vi "GetModuleReport (SubVI).vi"(8 "error in (no error)":errorcluster, 9 "Calibrated positions of fiducials [mm]":dbl[][](array[numeric]), 10 "ith Module":i32, 11 "Module Progress Report in":T1(array[cluster])) -> (0 "error out":errorcluster, 1 "MyCorners":dbl[][](array[numeric]), 2 "Array of ith module cluster fiducial mark positions":cluster{"X":dbl, "Y":dbl, "Z":dbl}[](array[cluster]), 3 "Module Progress Report out":T1(array[cluster]))   [LabVIEW 2016]
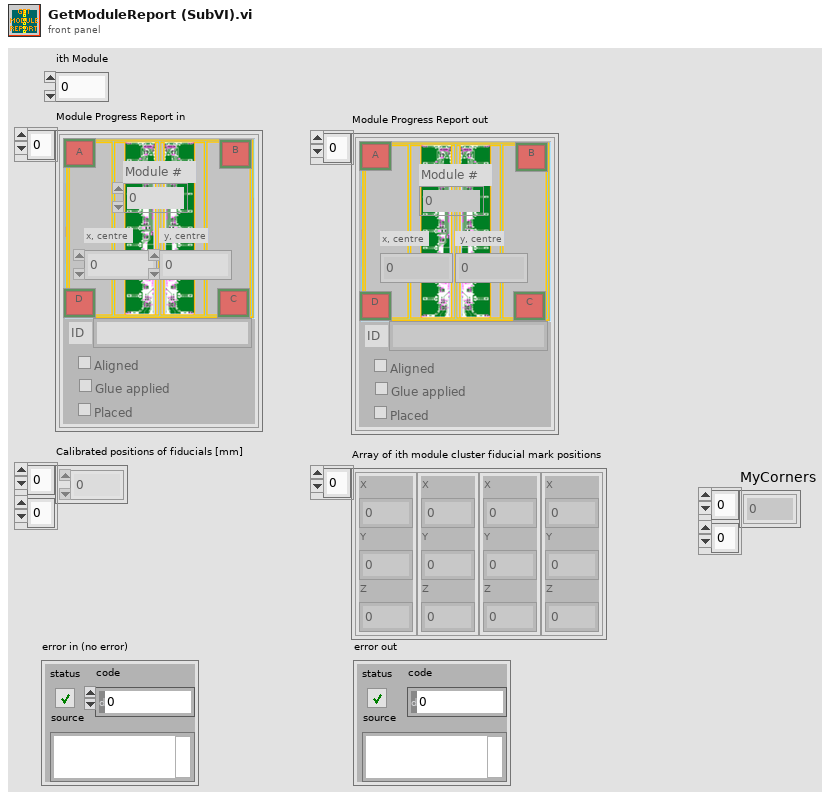
[diagram p1: front panel]
types:
  T1 = cluster{"B":bool, "A":bool, "D":bool, "C":bool, "ID":string, "Module #":i32, "x, centre":dbl, "y, centre":dbl, "Aligned":bool, "Glue applied":bool, "Placed":bool}[]
  T2 = cluster{"B":bool, "A":bool, "D":bool, "C":bool, "ID":string, "Module #":i32, "x, centre":dbl, "y, centre":dbl, "Aligned":bool, "Glue applied":bool, "Placed":bool}
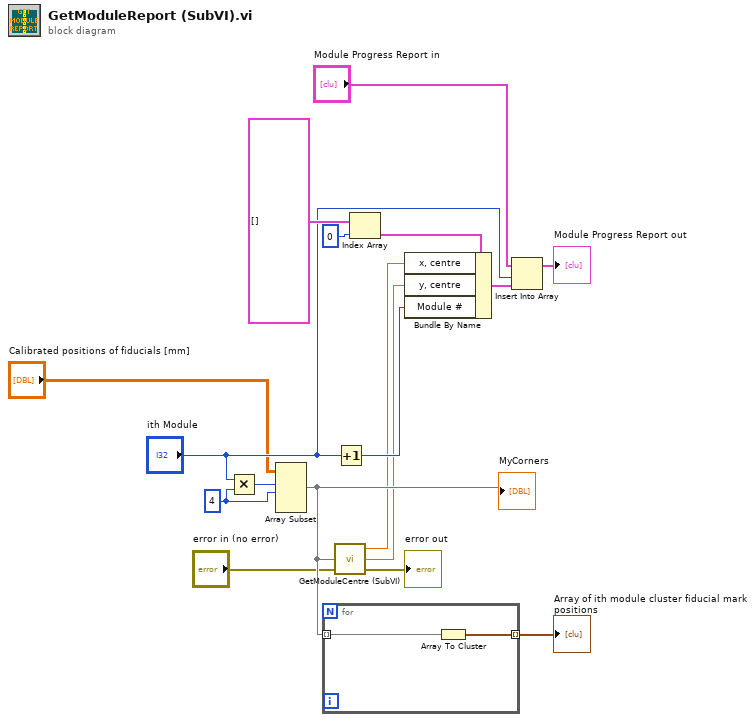
[diagram p0: block diagram]
diagram:
  w3 = 4 ("x")
  n1 = Multiply(x="ith Module", y=w3) -> (x*y=w2:i32)
  n2 = Array Subset(array="Calibrated positions of fiducials [mm]", index (row)=w2, length (row)=w3) -> (w13:dbl[][])  [unwired: 2 in]
  "MyCorners" <- w13
  n3 = for {
    tunnel: w13 -> [w18] mode=indexing
    tunnel: [w19] -> w4 mode=indexing
    n4 = Array To Cluster(array=w18) -> (cluster=w19:cluster{"[0]":dbl, "[1]":dbl, "[2]":dbl})
  }
  "Array of ith module cluster fiducial mark positions" <- w4
  n5 = call "GetModuleCentre (SubVI).vi"("error in (no error)"="error in (no error)", "4x3 Array of Fiducial Coordinates"=w13) -> ("error out"=→"error out":errorcluster, "y, centre"=w6:dbl, "x, centre"=w5:dbl)  [unwired: 1 in]
  n6 = Increment(x="ith Module") -> (x+1=w7:i32)
  n7 = Index Array(array=T1 [] ("Module Progress Report"), index=0) -> (element=w14:T2)
  n8 = Bundle By Name(cluster=w14, "x, centre"=w5, "y, centre"=w6, "Module #"=w7) -> (w17:T2)
  n9 = Insert Into Array(array="Module Progress Report in", index="ith Module", new element=w17) -> (→"Module Progress Report out":T1)
